vi "GlobalHum1.vi"() -> ()   [LabVIEW 2024]
panel:
  out "Hum1":dbl
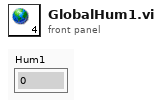
[diagram p1: front panel]
diagram:
